vi "Add Element to Control.vi"(6 "Default C++ Value (\"\")":string, 9 "Element Name":string, 10 "Cluster or Array":refnum<vi>, 11 "Abstract Param Writer in":refnum<class "Abstract Param Writer.lvclass">) -> (2 "Cluster or Array Dup":refnum<vi>, 3 "Abstract Param Writer out":refnum<class "Abstract Param Writer.lvclass">)   [LabVIEW 2014, in "Abstract Param Writer.lvclass"]
doc: "Adds a field to a cluster or array control.\n\nCopyright (c) 2021 Sze Howe Koh. This Source Code Form is subject to the terms of the Mozilla Public License, v. 2.0. If a copy of the MPL was not distributed with this file, You can obtain one at http://mozilla.org/MPL/2.0/."
uses:
  Abstract Param Writer.lvclass
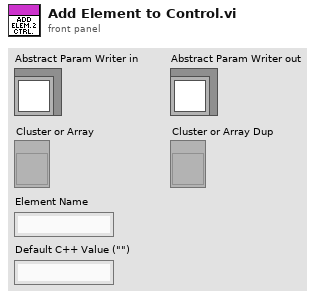
[diagram p1: front panel]
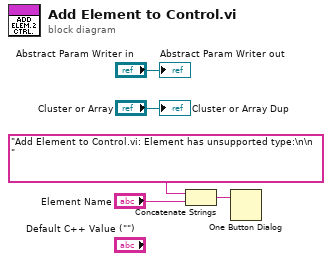
[diagram p0: block diagram]
diagram:
  n1 = Concatenate Strings("Add Element to Control.vi: Element has unsupported type:\n\n    ", "Element Name") -> (w1:string)
  n2 = One Button Dialog(message=w1) -> ()  [unwired: 1 in, 1 out]
  "Abstract Param Writer out" <- "Abstract Param Writer in"
  "Cluster or Array Dup" <- "Cluster or Array"
